vi "PH_GUI.set error GUI object.vi"(2 "GUI Refs.Device Error":refnum<vi>, 3 "error to set":errorcluster, 4 "Blinking (false)":bool, 5 "error in (no error)":errorcluster) -> (19 "error out":errorcluster)   [LabVIEW 2014, in "PH_Common.lvlib"]
doc: "Sets value and more for the referenced GUI object."
uses:
  PH_Common.lvlib
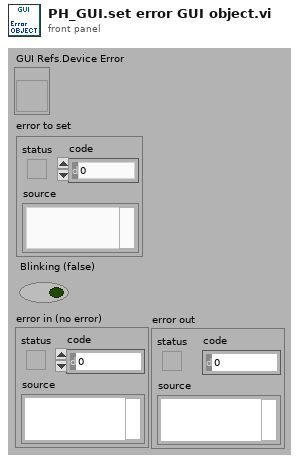
[diagram p1: front panel]
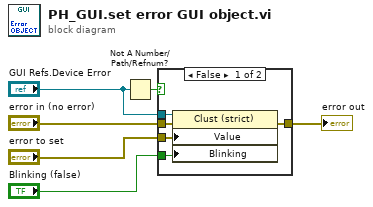
[diagram p0: block diagram]
diagram:
  n1 = Not A Number/Path/Refnum?(number/path/refnum="GUI Refs.Device Error") -> (NaN/Path/Refnum?=w5:bool)
  n2 = case shown="False" w5 {
    tunnel: "error in (no error)" -> [w11 w12]
    tunnel: [w10 w12] -> w6
    tunnel: "GUI Refs.Device Error" -> [w9 _]
    tunnel: "error to set" -> [w8 _]
    tunnel: "Blinking (false)" -> [w7 _]
    frame False {
      n3 = property class="Clust (strict)"(reference=w9, error in=w11, "Value"=w8, "Blinking"=w7) -> (error out=w10:errorcluster)  [unwired: 1 out]
    }
    frame True {
    }
  }
  "error out" <- w6
